vi "lvapi.vi"() -> ()   [LabVIEW 2018]
uses:
  <vilib>/MediaMongrels Ltd/WebSockets/WebSockets/WebSocket Server/WebSocket Server.lvclass
  C:/Program Files (x86)/National Instruments/LabVIEW 2018/vi.lib/MediaMongrels Ltd/WebSockets/WebSockets/WebSocket/WebSocket.lvclass
  <vilib>/MediaMongrels Ltd/WebSockets/Sockets/VISA TCP Listener/VISA TCP Listener.lvclass
panel:
  out "parsed data":cluster{"cmd":string, "data":string}
  in  "Command":string
  out "Received Data":string
  in  "Stop":bool
  in  "Send":bool
  in  "Data":string
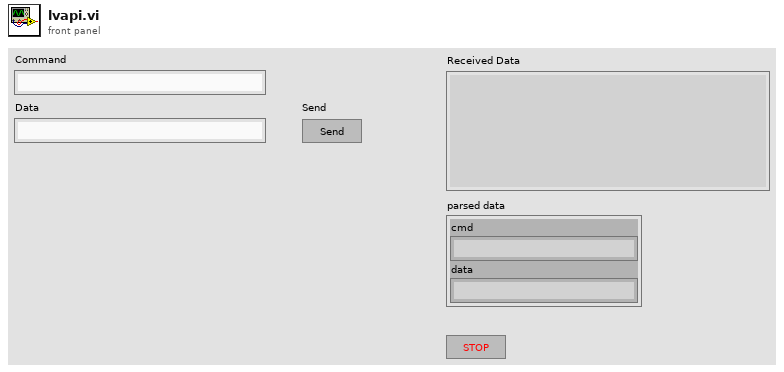
[diagram p1: front panel]
types:
  T1 = cluster{"cmd":string, "data":string, "dtype":string}
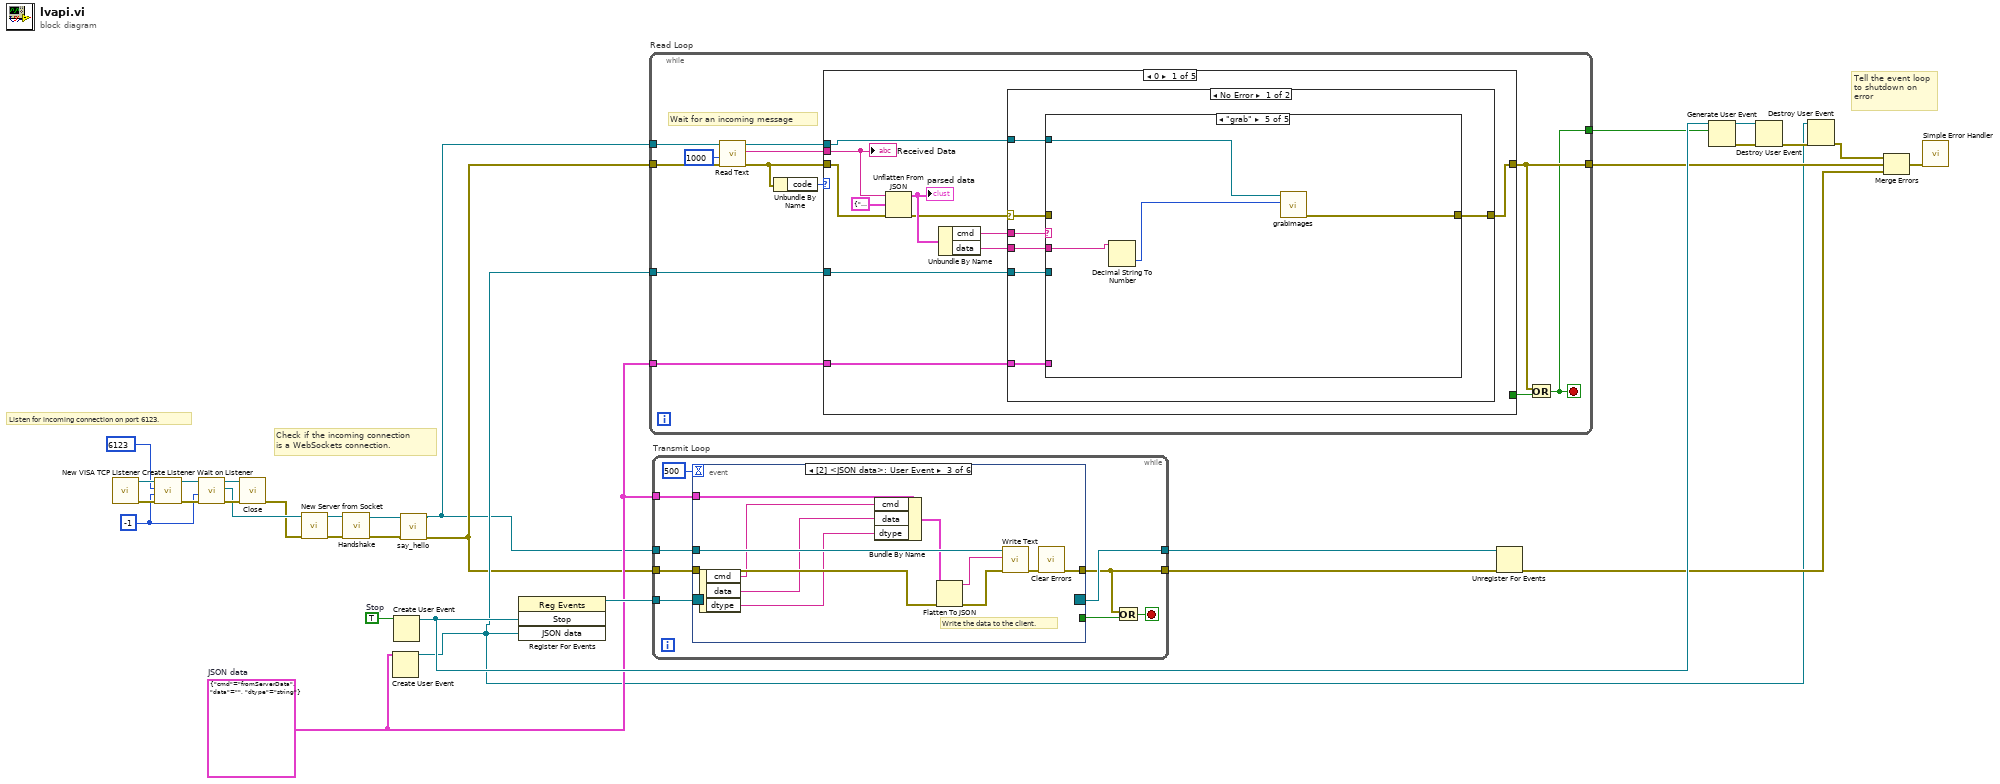
[diagram p0: block diagram]
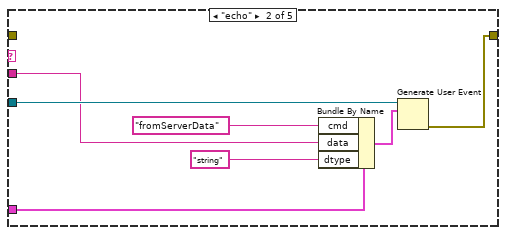
[diagram p3: hidden frame]
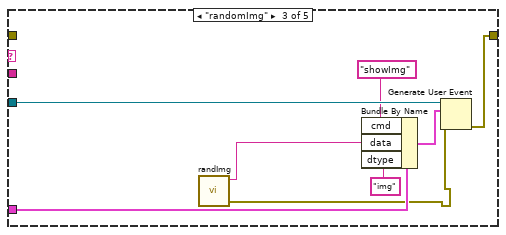
[diagram p4: hidden frame]
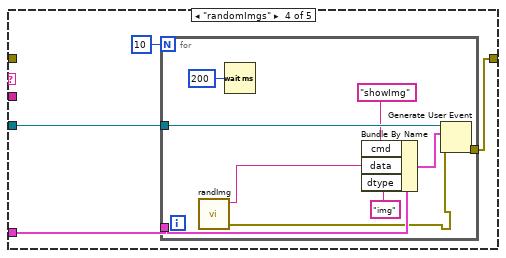
[diagram p5: hidden frame]
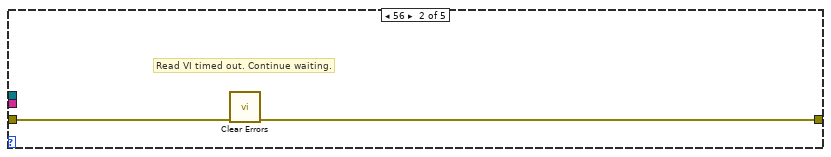
[diagram p7: hidden frame]
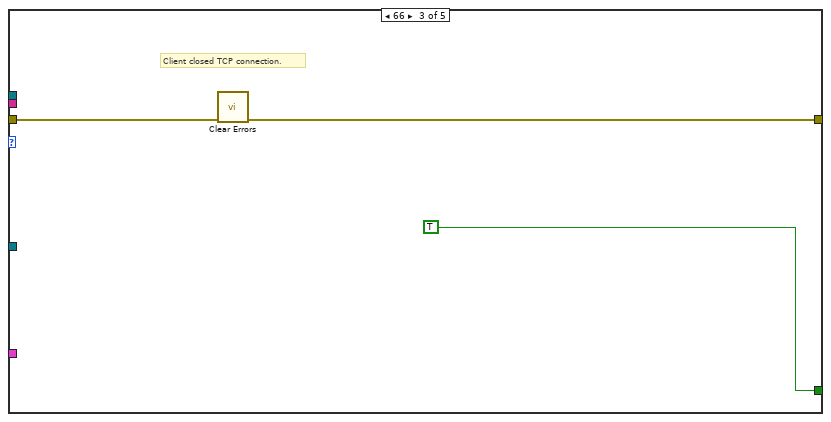
[diagram p8: hidden frame]
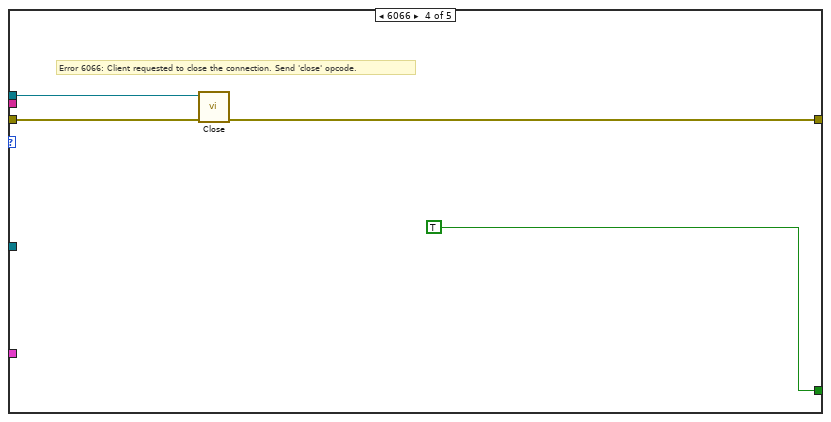
[diagram p9: hidden frame]
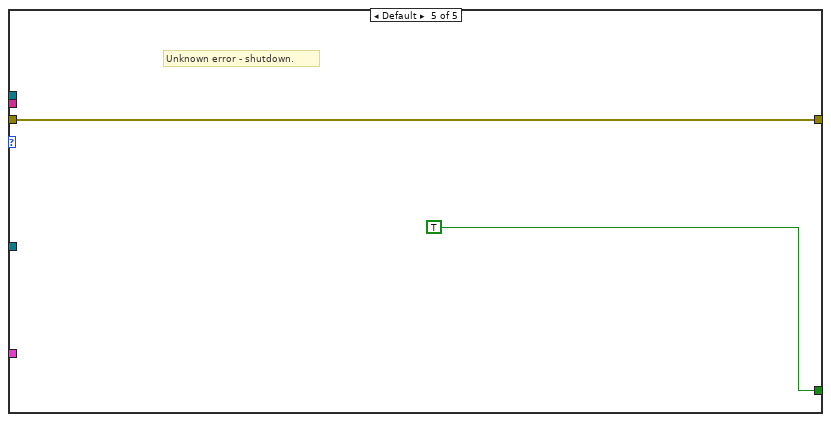
[diagram p10: hidden frame]
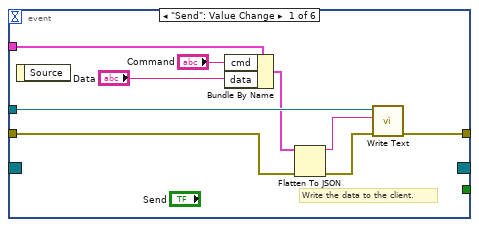
[diagram p11: hidden frame]
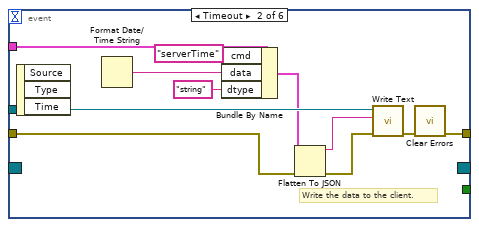
[diagram p12: hidden frame]
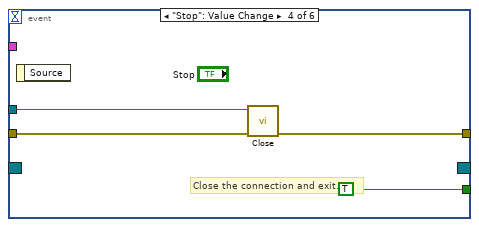
[diagram p13: hidden frame]
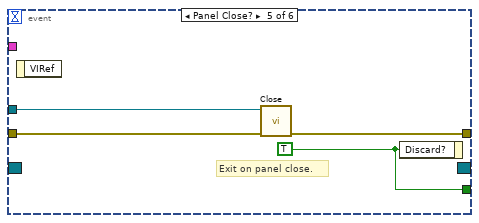
[diagram p14: hidden frame]
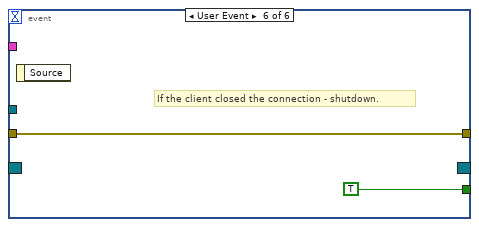
[diagram p15: hidden frame]
diagram:
  w8 = T1 {"cmd"="fromServerData", "data"="", "dtype"="string"}  # JSON data
  w30 = TRUE  # Stop
  w11 = -1 ("timeout ms (25000)")
  # "Tell the event loop to shutdown on error"
  # "Check if the incoming connection\nis a WebSockets connection."
  # "Listen for incoming connection on port 6123."
  n1 = call <vilib>:"New VISA TCP Listener.vi"() -> ("error out"=w17:errorcluster, "VISA TCP Listener out"=w18:refnum<class "VISA TCP Listener.lvclass">)  [unwired: 10 in]
  n2 = call-dynamic "Create Listener.vi"("error in (no error)"=w17, "timeout ms (5000)"=w11, "Port"=u16 6123 ("port"), "VISA TCP Listener in"=w18) -> ("error out"=w15:errorcluster, "VISA TCP Listener out"=w13:refnum<class "VISA TCP Listener.lvclass">)  [unwired: 6 in]
  n3 = call-dynamic "Wait on Listener.vi"("error in (no error)"=w15, "timeout ms (5000)"=w11, "VISA TCP Listener in"=w13) -> ("error out"=w16:errorcluster, "Socket out"=w10:refnum<class "Socket.lvclass">, "VISA TCP Listener out"=w14:refnum<class "VISA TCP Listener.lvclass">)  [unwired: 6 in]
  n4 = call-dynamic "Close.vi"("error in (no error)"=w16, "VISA TCP Listener in"=w14) -> ("error out"=w9:errorcluster)  [unwired: 9 in]
  n5 = call <vilib>:"New Server from Socket.vi"("error in (no error)"=w9, "Socket"=w10) -> ("error out"=w19:errorcluster, "WebSocket Server out"=w20:refnum<class "WebSocket Server.lvclass">)  [unwired: 8 in]
  n6 = call-dynamic "Handshake.vi"("error in (no error)"=w19, "WebSocket Connection in"=w20) -> ("error out"=w4:errorcluster, "WebSocket Connection out"=w2:refnum<class "WebSocket Server.lvclass">)  [unwired: 8 in]
  n7 = Create User Event(user event datatype=w8) -> (user event=w5:refnum<user-event>)  [unwired: 1 in, 1 out]
  n8 = Create User Event(user event datatype=w30) -> (user event=w28:refnum<user-event>)  [unwired: 1 in, 1 out]
  n9 = call "say_hello.vi"("error in (no error)"=w4, "WebSocket in"=w2) -> ("error out"=w3:errorcluster, "WebSocket out"=w1:refnum<class "WebSocket Server.lvclass">)  [unwired: 8 in]
  n10 = register-events(w28, w5) -> (reference out=w31:refnum<event-registration>)  [unwired: 2 in, 1 out]
  n11 = while "Read Loop" {
    tunnel: w1 -> [w43]
    tunnel: [w34] -> w27
    tunnel: [w36] -> w22
    tunnel: w3 -> [w37]
    tunnel: w5 -> [w33]
    tunnel: w8 -> [w32]
    stop <- w34 stop-if-true
    # "Wait for an incoming message"
    n12 = call-dynamic "Read Text.vi"("error in (no error)"=w37, "timeout ms (5000)"=1000 ("timeout ms (25000)"), "WebSocket in"=w43) -> ("error out"=w38:errorcluster, "Data"=w40:string, "WebSocket out"=w39:refnum<class "WebSocket Server.lvclass">)  [unwired: 6 in]
    n13 = Unbundle By Name(w38) -> ("code"=w41:i32)
    n14 = case shown="0" w41 {
      tunnel: w40 -> [w53 _ _ _ _]
      tunnel: [_ _ TRUE TRUE TRUE] -> w35
      tunnel: w39 -> [w44 _ _ w104 _]
      tunnel: w38 -> [w52 w97 w99 w102 w105]
      tunnel: [w49 w96 w98 w101 w105] -> w36
      tunnel: w33 -> [w45 _ _ _ _]
      tunnel: w32 -> [w46 _ _ _ _]
      frame 0 {
        n15 = Unflatten From JSON(JSON string=w53, type and defaults=cluster{"cmd":string, "data":string} {"cmd"="", "data"=""}, error in (no error)=w52) -> (value=w51:cluster{"cmd":string, "data":string}, error out=w50:errorcluster)  [unwired: 4 in]
        "parsed data" <- w51
        n16 = Unbundle By Name(w51) -> ("cmd"=w48:string, "data"=w47:string)
        n17 = case shown="No Error" w50 {
          selector: w50 -> [w59 w95]
          tunnel: [w60 w95] -> w49
          tunnel: w48 -> [w61 _]
          tunnel: w47 -> [w58 _]
          tunnel: w46 -> [w57 _]
          tunnel: w45 -> [w56 _]
          tunnel: w44 -> [w55 _]
          frame No Error {
            n18 = case shown="\"grab\"" w61 {
              tunnel: [w62 w66 w74 w79 w93] -> w60
              tunnel: w59 -> [w62 _ _ _ _]
              tunnel: w58 -> [_ w64 _ _ w92]
              tunnel: w57 -> [_ w68 w76 w80 _]
              tunnel: w56 -> [_ w69 w77 w81 _]
              tunnel: w55 -> [_ _ _ _ w94]
              frame "False", Default {
              }
              frame "echo" {
                n19 = Bundle By Name(cluster=w68, "cmd"="fromServerData", "data"=w64, "dtype"="string") -> (w67:T1)
                n20 = Generate User Event(user event=w69, event data cluster=w67) -> (error out=w66:errorcluster)  [unwired: 2 in, 1 out]
              }
              frame "randomImg" {
                n21 = call "randImg.vi"() -> ("error out"=w71:errorcluster, "string out (base64-encoded)"=w70:string)  [unwired: 9 in, 1 out]
                n22 = Bundle By Name(cluster=w76, "cmd"="showImg", "data"=w70, "dtype"="img") -> (w75:T1)
                n23 = Generate User Event(user event=w77, event data cluster=w75, error in=w71) -> (error out=w74:errorcluster)  [unwired: 1 in, 1 out]
              }
              frame "randomImgs" {
                n24 = for {
                  N: 10 -> [_]
                  tunnel: w81 -> [w90]
                  tunnel: w80 -> [w89]
                  tunnel: [w87] -> w79
                  n25 = call "randImg.vi"() -> ("error out"=w84:errorcluster, "string out (base64-encoded)"=w83:string)  [unwired: 9 in, 1 out]
                  n26 = Wait (ms)(milliseconds to wait=u32 200) -> ()  [unwired: 1 out]
                  n27 = Bundle By Name(cluster=w89, "cmd"="showImg", "data"=w83, "dtype"="img") -> (w88:T1)
                  n28 = Generate User Event(user event=w90, event data cluster=w88, error in=w84) -> (error out=w87:errorcluster)  [unwired: 1 in, 1 out]
                }
              }
              frame "grab" {
                n29 = Decimal String To Number(string=w92) -> (number=w91:i32)  [unwired: 2 in, 1 out]
                n30 = call "grabImages.vi"("how many images"=w91, "WebSocket in"=w94) -> ("error out"=w93:errorcluster)  [unwired: 9 in]
              }
            }
          }
          frame Error {
          }
        }
        "Received Data" <- w53
      }
      frame 56 {
        # "Read VI timed out. Continue waiting."
        n31 = call <vilib>:"Clear Errors.vi"("error in (no error)"=w97) -> ("error out"=w96:errorcluster)  [unwired: 5 in, 1 out]
      }
      frame 66 {
        # "Client closed TCP connection."
        n32 = call <vilib>:"Clear Errors.vi"("error in (no error)"=w99) -> ("error out"=w98:errorcluster)  [unwired: 5 in, 1 out]
      }
      frame 6066 {
        # "Error 6066: Client requested to close the connection. Send 'close' opcode."
        n33 = call-dynamic "Close.vi"("error in (no error)"=w102, "WebSocket in"=w104) -> ("error out"=w101:errorcluster)  [unwired: 9 in]
      }
      frame Default {
        # "Unknown error - shutdown."
      }
    }
    n34 = Or(x=w36, y=w35) -> (x .or. y?=w34:bool)
  }
  n35 = while "Transmit Loop" {
    tunnel: w1 -> [w115]
    tunnel: w31 -> [w114]
    tunnel: [w113] -> w29
    tunnel: [w109] -> w23
    tunnel: w3 -> [w112]
    tunnel: w8 -> [w107]
    stop <- w110 stop-if-true
    n36 = event shown="[2] <JSON data>: User Event" {
      selector: w114 -> [_ _ _ _ _ _]
      dyn-events: [_ _ _ _ _ _] -> w113
      timeout: 500 -> [_ _ _ _ _ _]
      tunnel: w115 -> [w124 w135 w146 w149 w154 _]
      tunnel: [_ _ _ TRUE w153 TRUE] -> w111
      tunnel: [w123 w128 w140 w148 w152 w155] -> w109
      tunnel: w112 -> [w122 w133 w144 w147 w151 w155]
      tunnel: w107 -> [w116 w126 w139 _ _ _]
      event "Send": Value Change {
        # "Write the data to the client."
        n37 = event-data() -> ()  [unwired: 1 in, 1 out]
        n38 = Bundle By Name(cluster=w116, "cmd"="Command", "data"="Data") -> (w117:T1)
        n39 = Flatten To JSON(anything=w117, error in (no error)=w122) -> (JSON string=w119:string, 11:w121:errorcluster)  [unwired: 1 in]
        n40 = call-dynamic "Write Text.vi"("error in (no error)"=w121, "String Data"=w119, "WebSocket in"=w124) -> ("error out"=w123:errorcluster)  [unwired: 7 in, 1 out]
      }
      event Timeout {
        # "Write the data to the client."
        n41 = event-data() -> ()  [unwired: 1 in, 3 out]
        n42 = Format Date/Time String() -> (date/time string=w127:string)  [unwired: 3 in]
        n43 = Bundle By Name(cluster=w126, "cmd"="serverTime" ("Command 2"), "data"=w127, "dtype"="string") -> (w129:T1)
        n44 = Flatten To JSON(anything=w129, error in (no error)=w133) -> (JSON string=w130:string, 11:w132:errorcluster)  [unwired: 1 in]
        n45 = call-dynamic "Write Text.vi"("error in (no error)"=w132, "String Data"=w130, "WebSocket in"=w135) -> ("error out"=w134:errorcluster)  [unwired: 7 in, 1 out]
        n46 = call <vilib>:"Clear Errors.vi"("error in (no error)"=w134) -> ("error out"=w128:errorcluster)  [unwired: 5 in, 1 out]
      }
      event User Event {
        # "Write the data to the client."
        n47 = event-data() -> ("cmd"=w138:string, "data"=w137:string, "dtype"=w136:string)  [unwired: 1 in]
        n48 = Bundle By Name(cluster=w139, "cmd"=w138, "data"=w137, "dtype"=w136) -> (w141:T1)
        n49 = Flatten To JSON(anything=w141, error in (no error)=w144) -> (JSON string=w142:string, 11:w143:errorcluster)  [unwired: 1 in]
        n50 = call-dynamic "Write Text.vi"("error in (no error)"=w143, "String Data"=w142, "WebSocket in"=w146) -> ("error out"=w145:errorcluster)  [unwired: 7 in, 1 out]
        n51 = call <vilib>:"Clear Errors.vi"("error in (no error)"=w145) -> ("error out"=w140:errorcluster)  [unwired: 5 in, 1 out]
      }
      event "Stop": Value Change {
        # "Close the connection and exit."
        n52 = event-data() -> ()  [unwired: 1 in, 1 out]
        n53 = call-dynamic "Close.vi"("error in (no error)"=w147, "WebSocket in"=w149) -> ("error out"=w148:errorcluster)  [unwired: 9 in]
      }
      event Panel Close? {
        w153 = TRUE ("Discard?")
        # "Exit on panel close."
        n54 = event-data() -> ()  [unwired: 1 in, 1 out]
        n55 = call-dynamic "Close.vi"("error in (no error)"=w151, "WebSocket in"=w154) -> ("error out"=w152:errorcluster)  [unwired: 9 in]
        n56 = event-data("Discard?"=w153) -> ()  [unwired: 1 in, 1 out]
      }
      event User Event {
        # "If the client closed the connection - shutdown."
        n57 = event-data() -> ()  [unwired: 1 in, 1 out]
      }
    }
    n58 = Or(x=w109, y=w111) -> (x .or. y?=w110:bool)
  }
  n59 = Unregister For Events(event registration refnum=w29, error in=w23) -> (error out=w21:errorcluster)
  n60 = Generate User Event(user event=w28, event data cluster=w27) -> (user event out=w26:refnum<user-event>, error out=w25:errorcluster)  [unwired: 2 in]
  n61 = Destroy User Event(user event=w26, error in=w25) -> (error out=w7:errorcluster)
  n62 = Destroy User Event(user event=w5, error in=w7) -> (error out=w6:errorcluster)
  n63 = Merge Errors(w6, w22, w21) -> (w24:errorcluster)
  n64 = call <vilib>:"Simple Error Handler.vi"("error in (no error)"=w24) -> ()  [unwired: 4 in, 5 out]
